vi "programa 5.vi"() -> ()   [LabVIEW 2011]
panel:
  out "Personas":dbl
  in  "Planta":u16(ring) items=["Planta #1", "Planta #2", "Planta #3"]
  out "A/C":bool
  out "temperatura":i32(slide) scale=0.0..60.0
  # "Se genera la temp entre 1-60,\nse selecciona la planta usando el menu ring,\nluego se genera el numero de personas entre 1-50"
  # "Planta 1 si hay mas de 25 personas y la temperatura \nes mayor a 22 se enciende el A/C\n\nPlanta 2 si ahy mas de 30 personas y la temperatura\nes mayor a 27 se enciende el A/C\n\nPlanta 3 si ahy mas de 20 personas y la temperatura\nes mayor a 29 se enciende el A/C"
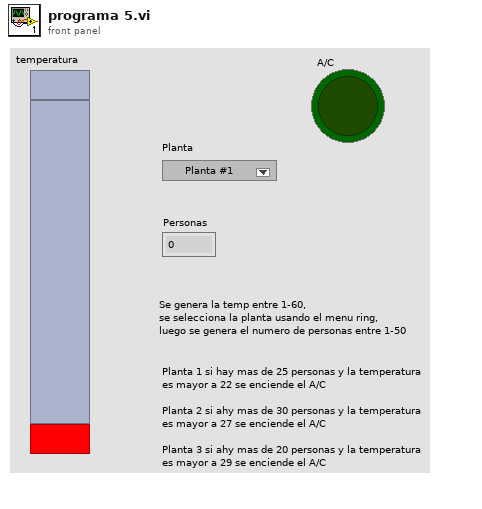
[diagram p1: front panel]
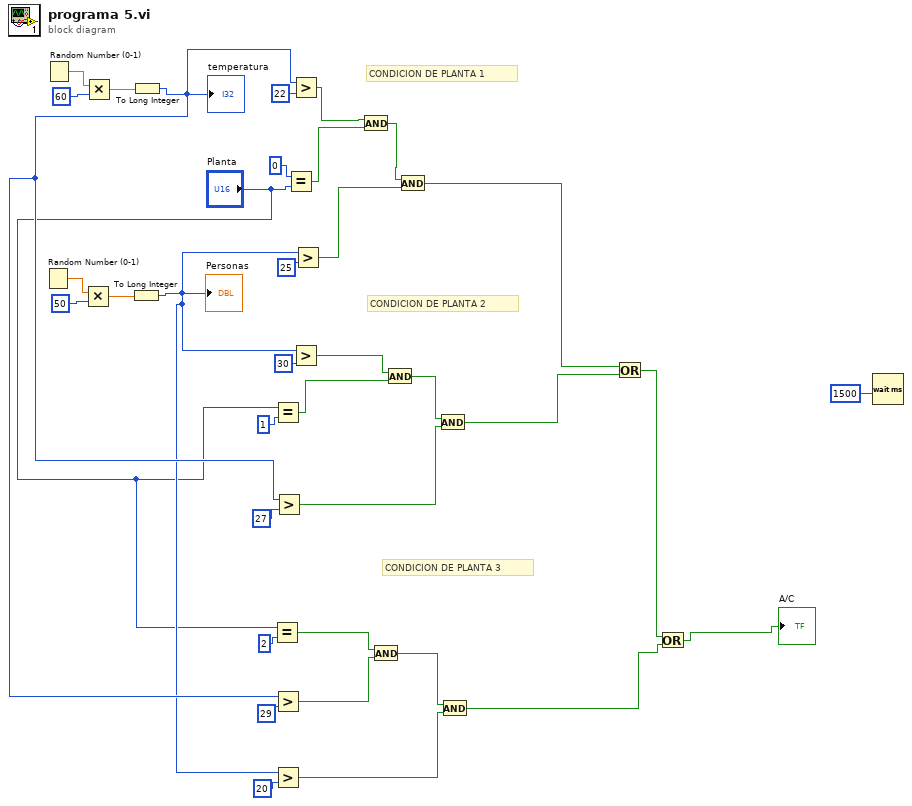
[diagram p0: block diagram]
diagram:
  # "CONDICION DE PLANTA 3"
  # "CONDICION DE PLANTA 2"
  # "CONDICION DE PLANTA 1"
  n1 = Random Number (0-1)() -> (number: 0 to 1=w31:dbl)
  n2 = Random Number (0-1)() -> (number: 0 to 1=w36:dbl)
  n3 = Multiply(x=w31, y=50) -> (x*y=w33:dbl)
  n4 = Multiply(x=w36, y=60) -> (x*y=w34:dbl)
  n5 = To Long Integer(number=w33) -> (32bit integer=w14:i32)
  "Personas" <- w14
  n6 = To Long Integer(number=w34) -> (32bit integer=w16:i32)
  "temperatura" <- w16
  n7 = Equal?(x="Planta", y=2) -> (x = y?=w10:bool)
  n8 = Equal?(x="Planta", y=1) -> (x = y?=w18:bool)
  n9 = Greater?(x=w16, y=29) -> (0:w9:bool)
  n10 = Greater?(x=w14, y=20) -> (0:w7:bool)
  n11 = Greater?(x=w16, y=27) -> (0:w17:bool)
  n12 = Equal?(x=0, y="Planta") -> (x = y?=w27:bool)
  n13 = Greater?(x=w16, y=22) -> (0:w26:bool)
  n14 = Greater?(x=w14, y=30) -> (0:w19:bool)
  n15 = Greater?(x=w14, y=25) -> (0:w25:bool)
  n16 = And(x=w26, y=w27) -> (x .and. y?=w24:bool)
  n17 = And(x=w10, y=w9) -> (x .and. y?=w8:bool)
  n18 = And(x=w19, y=w18) -> (x .and. y?=w20:bool)
  n19 = And(x=w24, y=w25) -> (x .and. y?=w6:bool)
  n20 = And(x=w20, y=w17) -> (x .and. y?=w5:bool)
  n21 = And(x=w8, y=w7) -> (x .and. y?=w3:bool)
  n22 = Or(x=w6, y=w5) -> (x .or. y?=w4:bool)
  n23 = Or(x=w4, y=w3) -> (x .or. y?=→"A/C":bool)
  n24 = Wait (ms)(milliseconds to wait=1500) -> ()  [unwired: 1 out]
